vi "AdvancingChangeField.vi"() -> ()   [LabVIEW 2019]
panel:
  in  "Boolean":bool
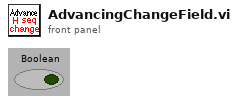
[diagram p1: front panel]
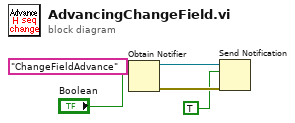
[diagram p0: block diagram]
diagram:
  n1 = Obtain Notifier(name (unnamed)="ChangeFieldAdvance", notification data type="Boolean") -> (notifier out=w4:refnum<notifier>, error out=w3:errorcluster)  [unwired: 2 in, 1 out]
  n2 = Send Notification(notification=TRUE, notifier=w4, error in (no error)=w3) -> ()  [unwired: 2 out]
